vi "onTestDiscovery.vi"(8 "error in (no error)":errorcluster, 11 "Test Runner in":refnum<class "Test Runner.lvclass">) -> (0 "error out":errorcluster, 2 "Tests VIs":path[](array[path]), 3 "Test Runner out":refnum<class "Test Runner.lvclass">)   [LabVIEW 2013, in "Caraya.lvlib" / "Test Runner.lvclass"]
uses:
  Test Runner.lvclass
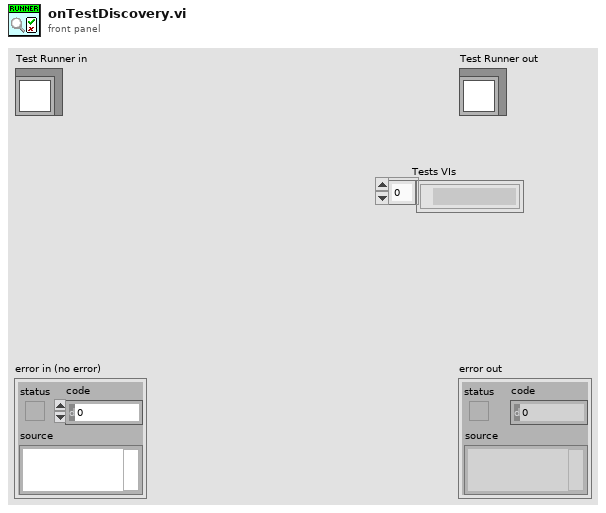
[diagram p1: front panel]
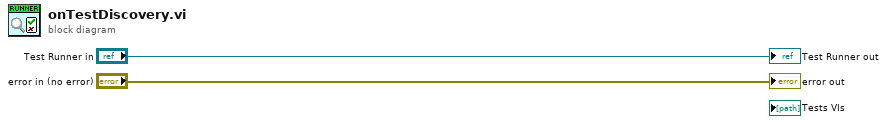
[diagram p0: block diagram]
diagram:
  "error out" <- "error in (no error)"
  "Test Runner out" <- "Test Runner in"
